vi "Swerve System Auton (SubVI).vi"(0 "Wheel Angle":T3, 5 "Wheel Power":T2, 11 "moduleAbsoluteAngles":T1) -> (1 "RightFrontWheelPowerDesired":dbl, 2 "LeftFrontWheelPowerDesired":dbl, 3 "LeftRearWheelPowerDesired":dbl, 4 "RightRearWheelPowerDesired":dbl, 6 "rightFrontAngleError":dbl, 8 "leftFrontAngleError":dbl, 10 "leftRearAngleError":dbl, 15 "rightRearAngleError":dbl)   [LabVIEW 2020]
uses:
  TypeDefs/WheelAngleDesired.ctl
  TypeDefs/WheelPowerDesired.ctl
panel:
  out "invertSpeedRightRear":bool
  out "invertSpeedLeftRear":bool
  out "invertSpeedLeftFront":bool
  out "invertSpeedRightFront":bool
  in  "Hysteresis (deg)":dbl=10.0
  in  "Zero Wheels":bool
  # "Inputs"
  # "Process Variables"
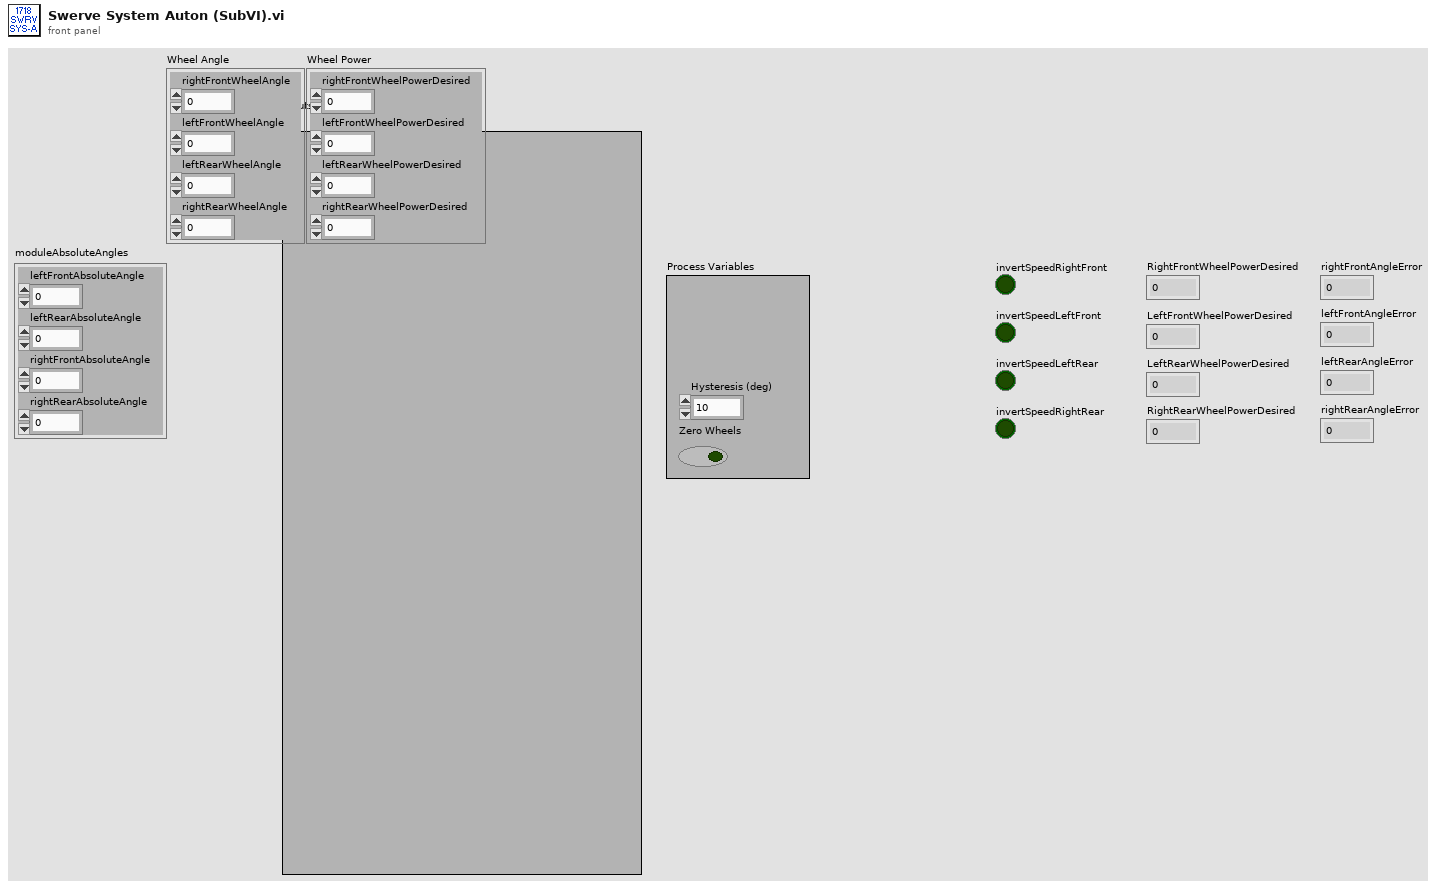
[diagram p1: front panel]
types:
  T1 = cluster{"leftFrontAbsoluteAngle":dbl, "leftRearAbsoluteAngle":dbl, "rightFrontAbsoluteAngle":dbl, "rightRearAbsoluteAngle":dbl}
  T2 = typedef "WheelPowerDesired.ctl" = cluster{"rightFrontWheelPowerDesired":dbl, "leftFrontWheelPowerDesired":dbl, "leftRearWheelPowerDesired":dbl, "rightRearWheelPowerDesired":dbl}
  T3 = typedef "WheelAngleDesired.ctl" = cluster{"rightFrontWheelAngle":dbl, "leftFrontWheelAngle":dbl, "leftRearWheelAngle":dbl, "rightRearWheelAngle":dbl}
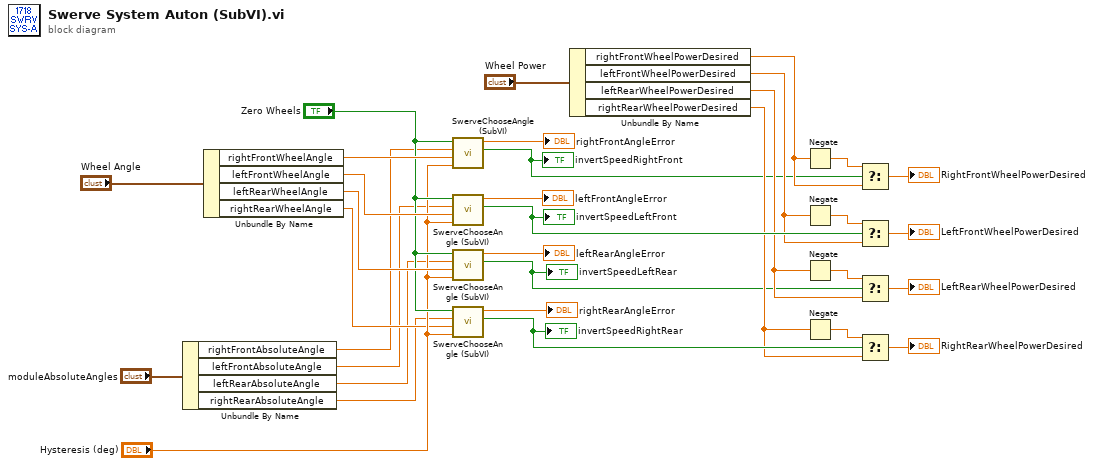
[diagram p0: block diagram]
diagram:
  n1 = Unbundle By Name("moduleAbsoluteAngles") -> ("rightFrontAbsoluteAngle"=w4:dbl, "leftFrontAbsoluteAngle"=w3:dbl, "leftRearAbsoluteAngle"=w2:dbl, "rightRearAbsoluteAngle"=w1:dbl)
  n2 = Unbundle By Name("Wheel Angle") -> ("rightFrontWheelAngle"=w31:dbl, "leftFrontWheelAngle"=w30:dbl, "leftRearWheelAngle"=w29:dbl, "rightRearWheelAngle"=w18:dbl)
  n3 = call "SwerveChooseAngle (SubVI).vi"("Hysteresis (deg)"="Hysteresis (deg)", "Goal Angle (deg)"=w31, "Current Angle (deg)"=w4, "Zero Wheels"="Zero Wheels") -> ("Invert Speed Motor"=w12:bool, "Angular Distance"=→"rightFrontAngleError":dbl)  [unwired: 5 in, 1 out]
  "invertSpeedRightFront" <- w12
  n4 = call "SwerveChooseAngle (SubVI).vi"("Hysteresis (deg)"="Hysteresis (deg)", "Goal Angle (deg)"=w30, "Current Angle (deg)"=w3, "Zero Wheels"="Zero Wheels") -> ("Invert Speed Motor"=w20:bool, "Angular Distance"=→"leftFrontAngleError":dbl)  [unwired: 5 in, 1 out]
  "invertSpeedLeftFront" <- w20
  n5 = call "SwerveChooseAngle (SubVI).vi"("Hysteresis (deg)"="Hysteresis (deg)", "Goal Angle (deg)"=w29, "Current Angle (deg)"=w2, "Zero Wheels"="Zero Wheels") -> ("Invert Speed Motor"=w13:bool, "Angular Distance"=→"leftRearAngleError":dbl)  [unwired: 5 in, 1 out]
  "invertSpeedLeftRear" <- w13
  n6 = call "SwerveChooseAngle (SubVI).vi"("Hysteresis (deg)"="Hysteresis (deg)", "Goal Angle (deg)"=w18, "Current Angle (deg)"=w1, "Zero Wheels"="Zero Wheels") -> ("Invert Speed Motor"=w19:bool, "Angular Distance"=→"rightRearAngleError":dbl)  [unwired: 5 in, 1 out]
  "invertSpeedRightRear" <- w19
  n7 = Unbundle By Name("Wheel Power") -> ("rightFrontWheelPowerDesired"=w17:dbl, "leftFrontWheelPowerDesired"=w16:dbl, "leftRearWheelPowerDesired"=w15:dbl, "rightRearWheelPowerDesired"=w14:dbl)
  n8 = Negate(x=w17) -> (-x=w33:dbl)
  n9 = Negate(x=w16) -> (-x=w25:dbl)
  n10 = Negate(x=w15) -> (-x=w24:dbl)
  n11 = Negate(x=w14) -> (-x=w21:dbl)
  n12 = Select(t=w33, s=w12, f=w17) -> (s? t:f=→"RightFrontWheelPowerDesired":dbl)
  n13 = Select(t=w25, s=w20, f=w16) -> (s? t:f=→"LeftFrontWheelPowerDesired":dbl)
  n14 = Select(t=w24, s=w13, f=w15) -> (s? t:f=→"LeftRearWheelPowerDesired":dbl)
  n15 = Select(t=w21, s=w19, f=w14) -> (s? t:f=→"RightRearWheelPowerDesired":dbl)
